vi "UIRef.vi"(8 "error in":errorcluster, 11 "node in":refnum<class "Run VI Node.lvclass">) -> (0 "error out":errorcluster, 2 "VI refnum":refnum<vi>, 3 "node out":refnum<class "Run VI Node.lvclass">)   [LabVIEW 2014, in "Run VI Node.lvclass"]
doc: "Stores the static reference to the UI of the node."
uses:
  Run VI Node.lvclass
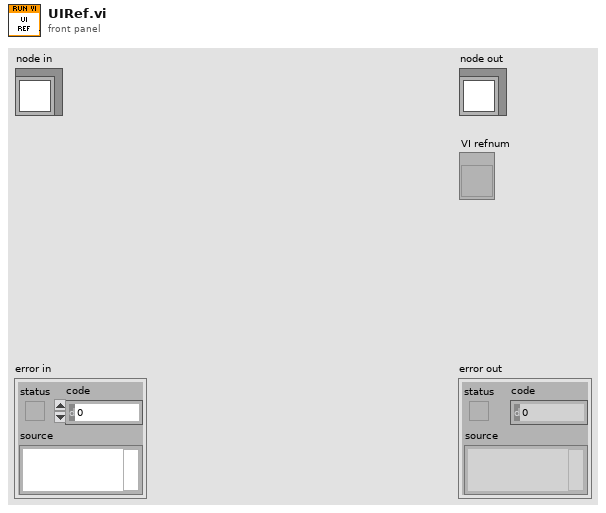
[diagram p1: front panel]
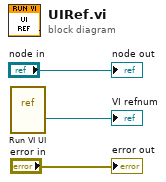
[diagram p0: block diagram]
diagram:
  n1 = vi-ref "Run VI UI.vi"() -> (→"VI refnum":refnum<vi>)
  "error out" <- "error in"
  "node out" <- "node in"
